vi "Reverse Polarity - Under Construction.vi"() -> ()   [LabVIEW 2020]
uses:
  <instrlib>/CAEN PSM/CAEN PSM.lvlib
  <vilib>/Utility/error.llb/DialogType.ctl
panel:
  in  "End Reverse Polarity":bool
  in  "Fast Ramp-up Speed\n(typically 50V/s)":dbl=250.0
  in  "Slow Ramp-up Speed\n(typically 10V/s)":dbl=10.0
  in  "Stop Voltage [V]\n(typically 3200V)":dbl=3200.0
  in  "Start Voltage [V]\n(typically 2000V)":dbl=1000.0
  in  "Current Theshold [uA]\n(typically 1uA)":dbl=1.0
  out "Polarity is set incorrectly if red":bool
  out "Power Trip":bool
  in  "VISA Refnum in":refnum<visa-resource-name>
  out "Voltage Ch 1":dbl
  out "Voltage Ch 0":dbl
  out "Current Ch 1":dbl
  out "Current Ch 0":dbl
  out "Performing Trip Tests":bool
  out "Test Is Running (Red)\nTest Is Stopped (Green)":bool
  in  "Start":bool
  # "Reverse Polarity Program 8/19/2021 This program will quickly ramp up to the specified \"Start Voltage\". It will then slowly increment to the stop voltage and recurrently check if the current is above threshold. If the current is above threshold, the program will wait unitl it drops below the threshold or timeout which occurs after 30min. The higher the threshold, the easier it will be for the power supply to trip. Therefore lower this threshold when dark current is very high. No check is done when initially ramping up, so make sure the \"Start Voltage\" is reasonably small. \n\nThere are two main error popups:\n\n\"Timeout Error\": Means you have to restart the power supply as the communication between the computer and labview is broken\n\n\"Unknown Error\": This will pop up every time you run, click \"continue\" and it will work."
  # "Red when power trips\nWhite when no power trip"
  # "Keep Going"
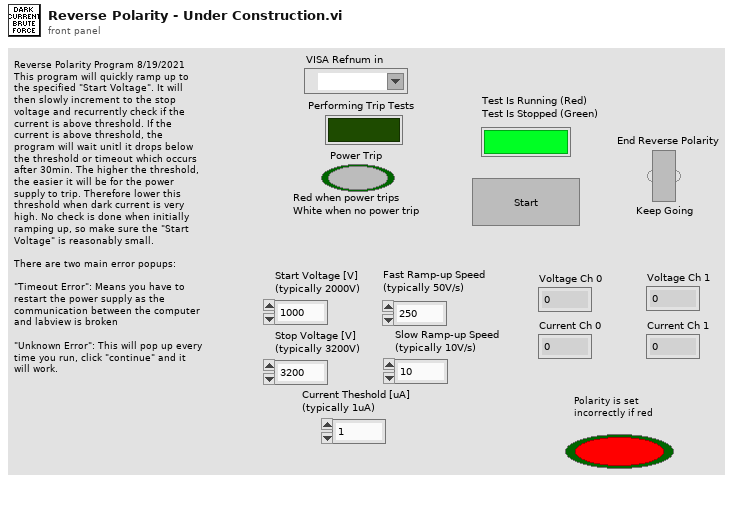
[diagram p1: front panel]
types:
  T1 = typedef "DialogType.ctl" = u16
  T2 = typedef "CAEN PSM.lvlib/BoardHandle.ctl" = cluster{"VISA resource name":refnum<visa-resource-name>, "Board address":i8, "NChannels":u8}
  T3 = cluster{"ON":bool, "RUP":bool, "RDW":bool, "OVC":bool, "OVV":bool, "UNV":bool, "MAXV":bool, "TRIP":bool, "OVP":bool, "OVT":bool, "DIS":bool, "KILL":bool, "ILK":bool, "NOCAL":bool}[]
  T4 = cluster{"ON":bool, "RUP":bool, "RDW":bool, "OVC":bool, "OVV":bool, "UNV":bool, "MAXV":bool, "TRIP":bool, "OVP":bool, "OVT":bool, "DIS":bool, "KILL":bool, "ILK":bool, "NOCAL":bool}
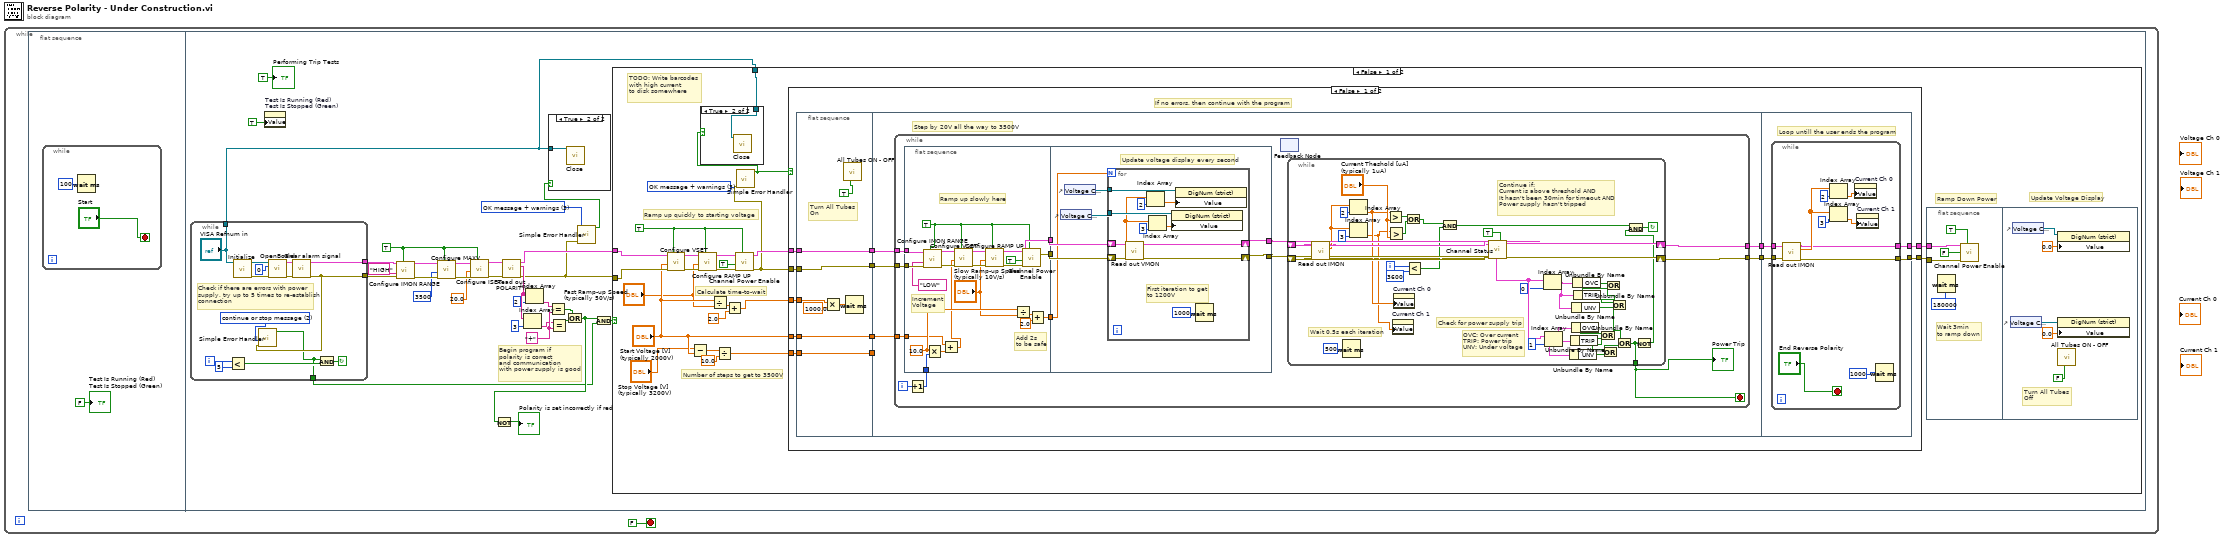
[diagram p0: block diagram]
diagram:
  n1 = while {
    stop <- FALSE stop-if-true
    n2 = flat-sequence {
      frame #0 {
        n3 = while {
          stop <- "Start" stop-if-true
          n4 = Wait (ms)(milliseconds to wait=u32 100) -> ()  [unwired: 1 out]
        }
        "Test Is Running (Red)\nTest Is Stopped (Green)" <- FALSE ("Start LED")
      }
      frame #1 {
        w7 = T1 3 items=["no dialog", "OK message", "continue or stop message", "OK message + warnings", "continue/stop + warnings"] ("type of dialog (OK msg:1)")
        w16 = "+"
        w27 = TRUE ("All Channels (F)")
        # "Begin program if\npolarity is correct\nand communication \nwith power supply is good"
        n5 = while {
          tunnel: [w45] -> w32
          tunnel: [w44] -> w12
          tunnel: [w38] -> w9
          tunnel: ["VISA Refnum in"] -> w5
          i -> [w42]
          stop <- w40 continue-if-true
          w43 = T1 2 items=["no dialog", "OK message", "continue or stop message", "OK message + warnings", "continue/stop + warnings"] ("type of dialog (OK msg:1)")
          # "Check if there are errors with power supply, try up to 5 times to re-establish connection"
          n6 = Less?(x=w42, y=5) -> (x < y?=w39:bool)
          n7 = call <instrlib>:"Initialize.vi"("VISA resource name"="VISA Refnum in") -> ("error out"=w48:errorcluster, "VISA resource name out"=w49:refnum<visa-resource-name>)  [unwired: 9 in]
          n8 = call <instrlib>:"OpenBoard.vi"("error in (no error)"=w48, "Board Address"=u8 0, "VISA resource name"=w49) -> ("error out"=w47:errorcluster, "BoardHandle"=w50:T2)  [unwired: 7 in]
          n9 = call <instrlib>:"Clear alarm signal.vi"("error in (no error)"=w47, "BoardHandle"=w50) -> ("error out"=w44:errorcluster, "BoardHandle out"=w45:T2)  [unwired: 8 in]
          n10 = call <vilib>:"Simple Error Handler.vi"("type of dialog (OK msg:1)"=w43, "error in (no error)"=w44) -> ("error?"=w38:bool)  [unwired: 3 in, 4 out]
          n11 = And(x=w38, y=w39) -> (x .and. y?=w40:bool)
        }
        n12 = property on="Test Is Running (Red)\nTest Is Stopped (Green)" class="Bool (strict)"("Value"=TRUE) -> ()  [unwired: 2 in, 2 out]
        n13 = call <instrlib>:"Configure IMON RANGE.vi"("All Channels (F)"=w27, "error in (no error)"=w12, "IMon range (LOW)"="HIGH", "BoardHandle"=w32) -> ("error out"=w30:errorcluster, "BoardHandle out"=w31:T2)  [unwired: 6 in]
        n14 = call <instrlib>:"Configure MAXV.vi"("All Channels (F)"=w27, "error in (no error)"=w30, "Voltage Max (0.0 V)"=u16 3500, "BoardHandle"=w31) -> ("error out"=w28:errorcluster, "BoardHandle out"=w29:T2)  [unwired: 6 in]
        n15 = call <instrlib>:"Configure ISET.vi"("All Channels (F)"=w27, "error in (no error)"=w28, "Current Limit (0.00 uA)"=sgl 20.0, "BoardHandle"=w29) -> ("error out"=w23:errorcluster, "BoardHandle out"=w24:T2)  [unwired: 6 in]
        n16 = call <instrlib>:"Read out POLARITY.vi"("error in (no error)"=w23, "BoardHandle"=w24) -> ("error out"=w8:errorcluster, "Polarity values"=w21:string[], "BoardHandle out"=w22:T2)  [unwired: 7 in]
        n17 = Index Array(array=w21, index=3) -> (element=w15:string)
        n18 = Index Array(array=w21, index=2) -> (element=w14:string)
        n19 = Equal?(x=w14, y=w16) -> (x = y?=w18:bool)
        n20 = Equal?(x=w15, y=w16) -> (x = y?=w17:bool)
        n21 = Or(x=w18, y=w17) -> (x .or. y?=w10:bool)
        n22 = Not(x=w10) -> (.not. x?=→"Polarity is set incorrectly if red":bool)
        n23 = call <vilib>:"Simple Error Handler.vi"("type of dialog (OK msg:1)"=w7, "error in (no error)"=w8) -> ("error?"=w6:bool)  [unwired: 3 in, 4 out]
        n24 = case shown="True" w6 {
          tunnel: w5 -> [_ w36]
          frame False {
          }
          frame True {
            n25 = call <instrlib>:"Close.vi"("VISA resource name"=w36) -> ()  [unwired: 10 in, 1 out]
          }
        }
        n26 = And(x=w10, y=w9) -> (x .and. y?=w11:bool)
        n27 = case shown="False" w11 {
          tunnel: w22 -> [w57 _]
          tunnel: w8 -> [w56 _]
          tunnel: w5 -> [w54 _]
          frame False {
            w58 = T1 3 items=["no dialog", "OK message", "continue or stop message", "OK message + warnings", "continue/stop + warnings"] ("type of dialog (OK msg:1)")
            w67 = TRUE ("All Channels (F)")
            # "Ramp up quickly to starting voltage"
            # "Number of steps to get to 3500V"
            # "Calculate time-to-wait"
            # "TODO: Write barcodes with high current\nto disk somewhere"
            # "Update Voltage Display"
            # "Ramp Down Power"
            n28 = call <instrlib>:"Configure VSET.vi"("All Channels (F)"=w67, "error in (no error)"=w56, "Voltage Level (0.0 V)"="Start Voltage [V]\n(typically 2000V)", "BoardHandle"=w57) -> ("error out"=w71:errorcluster, "BoardHandle out"=w70:T2)  [unwired: 6 in]
            n29 = Subtract(x="Stop Voltage [V]\n(typically 3200V)", y="Start Voltage [V]\n(typically 2000V)") -> (x-y=w62:dbl)
            n30 = call <instrlib>:"Configure RAMP UP.vi"("All Channels (F)"=w67, "error in (no error)"=w71, "Voltage ramp up (0 V/s)"="Fast Ramp-up Speed\n(typically 50V/s)", "BoardHandle"=w70) -> ("error out"=w72:errorcluster, "BoardHandle out"=w69:T2)  [unwired: 6 in]
            n31 = Divide(x="Start Voltage [V]\n(typically 2000V)", y="Fast Ramp-up Speed\n(typically 50V/s)") -> (x/y=w65:dbl)
            n32 = Divide(x=w62, y=10.0) -> (x/y=w60:dbl)
            n33 = Add(x=w65, y=2.0) -> (x+y=w63:dbl)
            n34 = call <instrlib>:"Channel Power Enable.vi"("All Channels (F)"=w67, "error in (no error)"=w72, "Enable (OFF)"=TRUE ("Boolean"), "BoardHandle"=w69) -> ("error out"=w59:errorcluster, "BoardHandle out"=w66:T2)  [unwired: 6 in]
            n35 = call <vilib>:"Simple Error Handler.vi"("type of dialog (OK msg:1)"=w58, "error in (no error)"=w59) -> ("error?"=w52:bool)  [unwired: 3 in, 4 out]
            n36 = case shown="True" w52 {
              tunnel: w54 -> [_ w212]
              frame False {
              }
              frame True {
                n37 = call <instrlib>:"Close.vi"("VISA resource name"=w212) -> ()  [unwired: 10 in, 1 out]
              }
            }
            n38 = case shown="False" w52 {
              tunnel: [w75 w211] -> w74
              tunnel: [w83 w210] -> w73
              tunnel: w66 -> [w82 w211]
              tunnel: w63 -> [w81 _]
              tunnel: w60 -> [w80 _]
              tunnel: w59 -> [w79 w210]
              tunnel: "Start Voltage [V]\n(typically 2000V)" -> [w78 _]
              frame False {
                # "If no errors, then continue with the program"
                n39 = flat-sequence {
                  tunnel: [w94] -> w87
                  tunnel: [w93] -> w86
                  tunnel: w82 -> [w94]
                  tunnel: w79 -> [w93]
                  tunnel: w81 -> [w90]
                  tunnel: [w89] -> w85
                  tunnel: w80 -> [w89]
                  tunnel: [w88] -> w84
                  tunnel: w78 -> [w88]
                  tunnel: w87 -> [w101]
                  tunnel: w86 -> [w100]
                  tunnel: w85 -> [w97]
                  tunnel: w84 -> [w96]
                  tunnel: [w99] -> w77
                  tunnel: [w98] -> w76
                  tunnel: [w195] -> w83
                  tunnel: [w196] -> w75
                  tunnel: w77 -> [w198]
                  tunnel: w76 -> [w197]
                  frame #0 {
                    # "Turn All Tubes \nOn"
                    n40 = Multiply(x=w90, y=1000.0) -> (x*y=w92:dbl)
                    n41 = call "All Tubes ON - OFF.vi"("Tubes ON/OFF"=TRUE ("Single Tube ON/OFF")) -> ()  [unwired: 11 in]
                    n42 = Wait (ms)(milliseconds to wait=w92) -> ()  [unwired: 1 out]
                  }
                  frame #1 {
                    # "Step by 20V all the way to 3500V"
                    n43 = while {
                      tunnel: w100 -> [w112]
                      tunnel: w101 -> [w111]
                      tunnel: [w104] -> w99
                      tunnel: [w105] -> w98
                      tunnel: w96 -> [w102]
                      i -> [w106]
                      stop <- w103 stop-if-true
                      n44 = flat-sequence {
                        tunnel: [w171] -> w114
                        tunnel: [w170] -> w113
                        tunnel: w107 -> [w168]
                        tunnel: w112 -> [w166]
                        tunnel: w111 -> [w167]
                        tunnel: [w158] -> w108
                        tunnel: w102 -> [w155]
                        tunnel: [w177] -> w110
                        tunnel: [w176] -> w109
                        tunnel: w108 -> [w180]
                        tunnel: w113 -> [w181]
                        tunnel: w114 -> [w182]
                        frame #0 {
                          w161 = 10.0 ("x")
                          w162 = TRUE ("All Channels (F)")
                          # "Ramp up slowly here"
                          # "Add 2s\nto be safe"
                          # "Increment\nVoltage"
                          n45 = call <instrlib>:"Configure IMON RANGE.vi"("All Channels (F)"=w162, "error in (no error)"=w166, "IMon range (LOW)"="LOW", "BoardHandle"=w167) -> ("error out"=w165:errorcluster, "BoardHandle out"=w164:T2)  [unwired: 6 in]
                          n46 = Multiply(x=w161, y=w168) -> (x*y=w157:dbl)
                          n47 = Add(x=w155, y=w157) -> (x+y=w156:dbl)
                          n48 = call <instrlib>:"Configure VSET.vi"("All Channels (F)"=w162, "error in (no error)"=w165, "Voltage Level (0.0 V)"=w156, "BoardHandle"=w164) -> ("error out"=w174:errorcluster, "BoardHandle out"=w173:T2)  [unwired: 6 in]
                          n49 = call <instrlib>:"Configure RAMP UP.vi"("All Channels (F)"=w162, "error in (no error)"=w174, "Voltage ramp up (0 V/s)"="Slow Ramp-up Speed\n(typically 10V/s)", "BoardHandle"=w173) -> ("error out"=w175:errorcluster, "BoardHandle out"=w172:T2)  [unwired: 6 in]
                          n50 = Divide(x=w161, y="Slow Ramp-up Speed\n(typically 10V/s)") -> (x/y=w159:dbl)
                          n51 = call <instrlib>:"Channel Power Enable.vi"("All Channels (F)"=w162, "error in (no error)"=w175, "Enable (OFF)"=TRUE ("Boolean"), "BoardHandle"=w172) -> ("error out"=w170:errorcluster, "BoardHandle out"=w171:T2)  [unwired: 6 in]
                          n52 = Add(x=w159, y=2.0) -> (x+y=w158:dbl)
                        }
                        frame #1 {
                          # "Update voltage display every second"
                          n53 = control-ref of="Voltage Ch 1"() -> (w178:refnum<vi>)
                          n54 = control-ref of="Voltage Ch 0"() -> (w179:refnum<vi>)
                          n55 = for {
                            N: w180 -> [_]
                            shift-right: [w191] -> w177
                            shift-left: w182 -> [w193]
                            shift-right: [w190] -> w176
                            shift-left: w181 -> [w192]
                            tunnel: w179 -> [w187]
                            tunnel: w178 -> [w185]
                            # "First iteration to get\nto 1200V"
                            n56 = call <instrlib>:"Read out VMON.vi"("error in (no error)"=w192, "BoardHandle"=w193) -> ("error out"=w190:errorcluster, "VMon values (V)"=w183:dbl[], "BoardHandle out"=w191:T2)  [unwired: 7 in]
                            n57 = Index Array(array=w183, index=2) -> (element=w188:dbl)
                            n58 = Index Array(array=w183, index=3) -> (element=w184:dbl)
                            n59 = property class="DigNum (strict)"(reference=w185, "Value"=w184) -> ()  [unwired: 1 in, 2 out]
                            n60 = property class="DigNum (strict)"(reference=w187, "Value"=w188) -> ()  [unwired: 1 in, 2 out]
                            n61 = Wait (ms)(milliseconds to wait=u32 1000) -> ()  [unwired: 1 out]
                          }
                        }
                      }
                      n62 = Increment(x=w106) -> (x+1=w107:i32)
                      n63 = feedback-in #1() -> ()  [unwired: 1 out]
                      n64 = feedback #1() -> ()  [unwired: 2 in]
                      n65 = while {
                        shift-right: [w120] -> w104
                        shift-left: w110 -> [w151]
                        shift-right: [w119] -> w105
                        shift-left: w109 -> [w150]
                        tunnel: [w115] -> w103
                        i -> [w144]
                        stop <- w116 continue-if-true
                        # "OVC: Over current\nTRIP: Power trip\nUNV: Under voltage"
                        # "Check for power supply trip"
                        # "Wait 0.5s each iteration"
                        # "Continue if:\nCurrent is above threshold AND\nIt hasn't been 30min for timeout AND\nPower supply hasn't tripped"
                        n66 = call <instrlib>:"Read out IMON.vi"("error in (no error)"=w150, "BoardHandle"=w151) -> ("error out"=w121:errorcluster, "IMon values (uA)"=w149:dbl[], "BoardHandle out"=w122:T2)  [unwired: 6 in, 1 out]
                        n67 = Wait (ms)(milliseconds to wait=u32 500) -> ()  [unwired: 1 out]
                        n68 = Index Array(array=w149, index=2) -> (element=w140:dbl)
                        n69 = Index Array(array=w149, index=3) -> (element=w139:dbl)
                        n70 = Greater?(x=w140, y="Current Theshold [uA]\n(typically 1uA)") -> (0:w147:bool)
                        n71 = Greater?(x=w139, y="Current Theshold [uA]\n(typically 1uA)") -> (0:w146:bool)
                        n72 = property on="Current Ch 1" class="DigNum (strict)"("Value"=w139) -> ()  [unwired: 2 in, 2 out]
                        n73 = property on="Current Ch 0" class="DigNum (strict)"("Value"=w140) -> ()  [unwired: 2 in, 2 out]
                        n74 = Or(x=w147, y=w146) -> (x .or. y?=w142:bool)
                        n75 = Less?(x=w144, y=3600) -> (x < y?=w141:bool)
                        n76 = And(x=w142, y=w141) -> (x .and. y?=w118:bool)
                        n77 = call <instrlib>:"Channel Status.vi"("All Channels (T)"=TRUE, "error in (no error)"=w121, "BoardHandle"=w122) -> ("error out"=w119:errorcluster, "Channel Status Array"=w138:T3, "BoardHandle out"=w120:T2)  [unwired: 5 in, 1 out]
                        n78 = Index Array(array=w138, index=0) -> (element=w130:T4)
                        n79 = Index Array(array=w138, index=1) -> (element=w126:T4)
                        n80 = Unbundle By Name(w126) -> ("UNV"=w125:bool)
                        n81 = Unbundle By Name(w126) -> ("TRIP"=w136:bool)
                        n82 = Unbundle By Name(w126) -> ("OVC"=w137:bool)
                        n83 = Unbundle By Name(w130) -> ("UNV"=w128:bool)
                        n84 = Unbundle By Name(w130) -> ("OVC"=w135:bool)
                        n85 = Unbundle By Name(w130) -> ("TRIP"=w134:bool)
                        n86 = Or(x=w137, y=w136) -> (x .or. y?=w123:bool)
                        n87 = Or(x=w123, y=w125) -> (x .or. y?=w124:bool)
                        n88 = Or(x=w135, y=w134) -> (x .or. y?=w129:bool)
                        n89 = Or(x=w129, y=w128) -> (x .or. y?=w127:bool)
                        n90 = Or(x=w127, y=w124) -> (x .or. y?=w115:bool)
                        n91 = Not(x=w115) -> (.not. x?=w117:bool)
                        n92 = And(x=w118, y=w117) -> (x .and. y?=w116:bool)
                      }
                      "Power Trip" <- w103
                    }
                  }
                  frame #2 {
                    # "Loop untill the user ends the program"
                    n93 = while {
                      tunnel: w198 -> [w204]
                      tunnel: w197 -> [w203]
                      tunnel: [w202] -> w196
                      tunnel: [w201] -> w195
                      stop <- "End Reverse Polarity" stop-if-true
                      n94 = call <instrlib>:"Read out IMON.vi"("error in (no error)"=w203, "BoardHandle"=w204) -> ("error out"=w201:errorcluster, "IMon values (uA)"=w205:dbl[], "BoardHandle out"=w202:T2)  [unwired: 6 in, 1 out]
                      n95 = Index Array(array=w205, index=2) -> (element=w199:dbl)
                      n96 = Index Array(array=w205, index=3) -> (element=w200:dbl)
                      n97 = property on="Current Ch 0" class="DigNum (strict)"("Value"=w199) -> ()  [unwired: 2 in, 2 out]
                      n98 = property on="Current Ch 1" class="DigNum (strict)"("Value"=w200) -> ()  [unwired: 2 in, 2 out]
                      n99 = Wait (ms)(milliseconds to wait=u32 1000) -> ()  [unwired: 1 out]
                    }
                  }
                }
              }
              frame True {
                # "An error occured, don't do the main program"
              }
            }
            n100 = flat-sequence {
              tunnel: w73 -> [w217]
              tunnel: w74 -> [w216]
              frame #0 {
                # "Wait 3min\nto ramp down"
                n101 = Wait (ms)(milliseconds to wait=u32 180000) -> ()  [unwired: 1 out]
                n102 = call <instrlib>:"Channel Power Enable.vi"("All Channels (F)"=TRUE, "error in (no error)"=w217, "Enable (OFF)"=FALSE, "BoardHandle"=w216) -> ()  [unwired: 6 in, 2 out]
              }
              frame #1 {
                # "Turn All Tubes \nOff"
                n103 = control-ref of="Voltage Ch 1"() -> (w221:refnum<vi>)
                n104 = control-ref of="Voltage Ch 0"() -> (w222:refnum<vi>)
                n105 = property class="DigNum (strict)"(reference=w222, "Value"=0.0) -> ()  [unwired: 1 in, 2 out]
                n106 = property class="DigNum (strict)"(reference=w221, "Value"=0.0) -> ()  [unwired: 1 in, 2 out]
                n107 = call "All Tubes ON - OFF.vi"("Tubes ON/OFF"=FALSE ("Single Tube ON/OFF")) -> ()  [unwired: 11 in]
              }
            }
          }
          frame True {
          }
        }
        "Performing Trip Tests" <- TRUE ("Performing Trip Tests")
      }
    }
  }
